vi "all-signals_counter-error-001.vi"() -> ()   [LabVIEW 2018]
uses:
  <vilib>/Platform/TimedLoop/XDataNode/timing_clust.ctl
  <vilib>/Platform/TimedLoop/XDataNode/nitl_modes.ctl
  <vilib>/Platform/TimedLoop/XDataNode/wakeup.ctl
  <vilib>/Analysis/baseanly.llb/Mean (DBL).vi
  <vilib>/platform/TimedLoop/XDataNode/XDataNode.xnode
  <vilib>/Analysis/NI_AALBase.lvlib
  <vilib>/Platform/TimedLoop/XDataNode/XDNodeRunTimeDep.lvlib
panel:
  in  "Clear Charts":bool
  in  "stop measurement (F)":bool caption="Stop measurements (F)"
  in  "Messzeit in ms":u32=100 min=10 max=1000 step=10
  in  "Tab Control":T1(tab)
  out "driving torque and counter":dynamicdata(graph)
  out "M_mech/N_motor":cluster{"Y":dbl[], "Y":dbl[]}[](graph)
  out "driving torque selected":dbl(graph)
  out "Motordrehzahl":dynamicdata(graph)
  out "Driving Torque gemittelt":dbl(graph)
  out "RPM and dn":dynamicdata(graph)
  out "Geschwindigkeit":dynamicdata(graph)
  out "Elektrische Leistung":waveform(dbl)(graph)
  out "RPM":dbl
  out "Bremsmoment":dynamicdata(graph)
  out "angular acc":dynamicdata(graph)
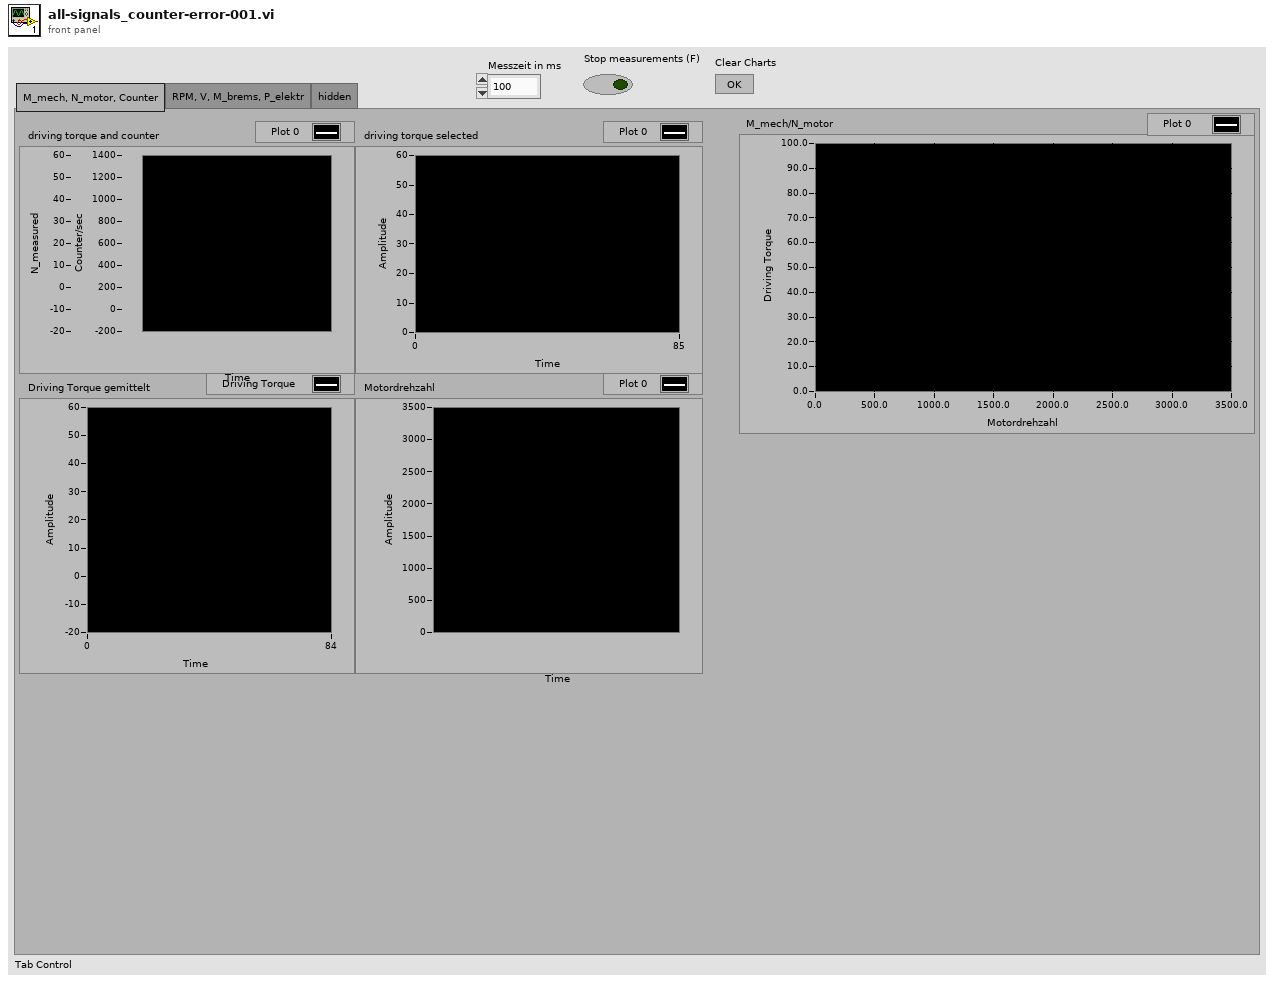
[diagram p1: front panel]
types:
  T1 = enum32{"M_mech, N_motor, Counter", "RPM, V, M_brems, P_elektr", "hidden"}
  T2 = typedef "XDNodeRunTimeDep.lvlib/timing_clust.ctl" = cluster{"Expected End [f-1]":u64, "Actual End [f-1]":u64, "Finished Late? [f-1]":bool, "Expected End [i-1]":u64, "Actual End [i-1]":u64, "Finished Late? [i-1]":bool, "Expected Start [i]":u64, "Actual Start [i]":u64, "Expected Start [f]":u64, "Actual Start [f]":u64, "Source Name":string, "Structure Name":string, "Period":i64, "Deadline":i64, "Offset":i64, "Start":i64, "Priority":i32, "Timeout":i32, "Mode":T3, "Wakeup Reason":T4, "Error":errorcluster, "Source Type":string, "Secondary Source Type":string, "Global End Time":u64, "Global Start Time":u64, "Frame Duration":u64, "Iteration Duration":u64, "Assigned CPU":i32, "I/O Scan Engine Mode":u32}
  T3 = typedef "XDNodeRunTimeDep.lvlib/nitl_modes.ctl" = enum32{"No Change", "Process missed periods, maintain original phase", "Discard missed periods, maintain original phase", "Process missed periods, ignore original phase", "Discard missed periods, ignore original phase"}
  T4 = typedef "XDNodeRunTimeDep.lvlib/wakeup.ctl" = enum32{"Normal", "Aborted", "Asynchronous wakeup", "Timing source error", "Timed loop error", "Timeout"}
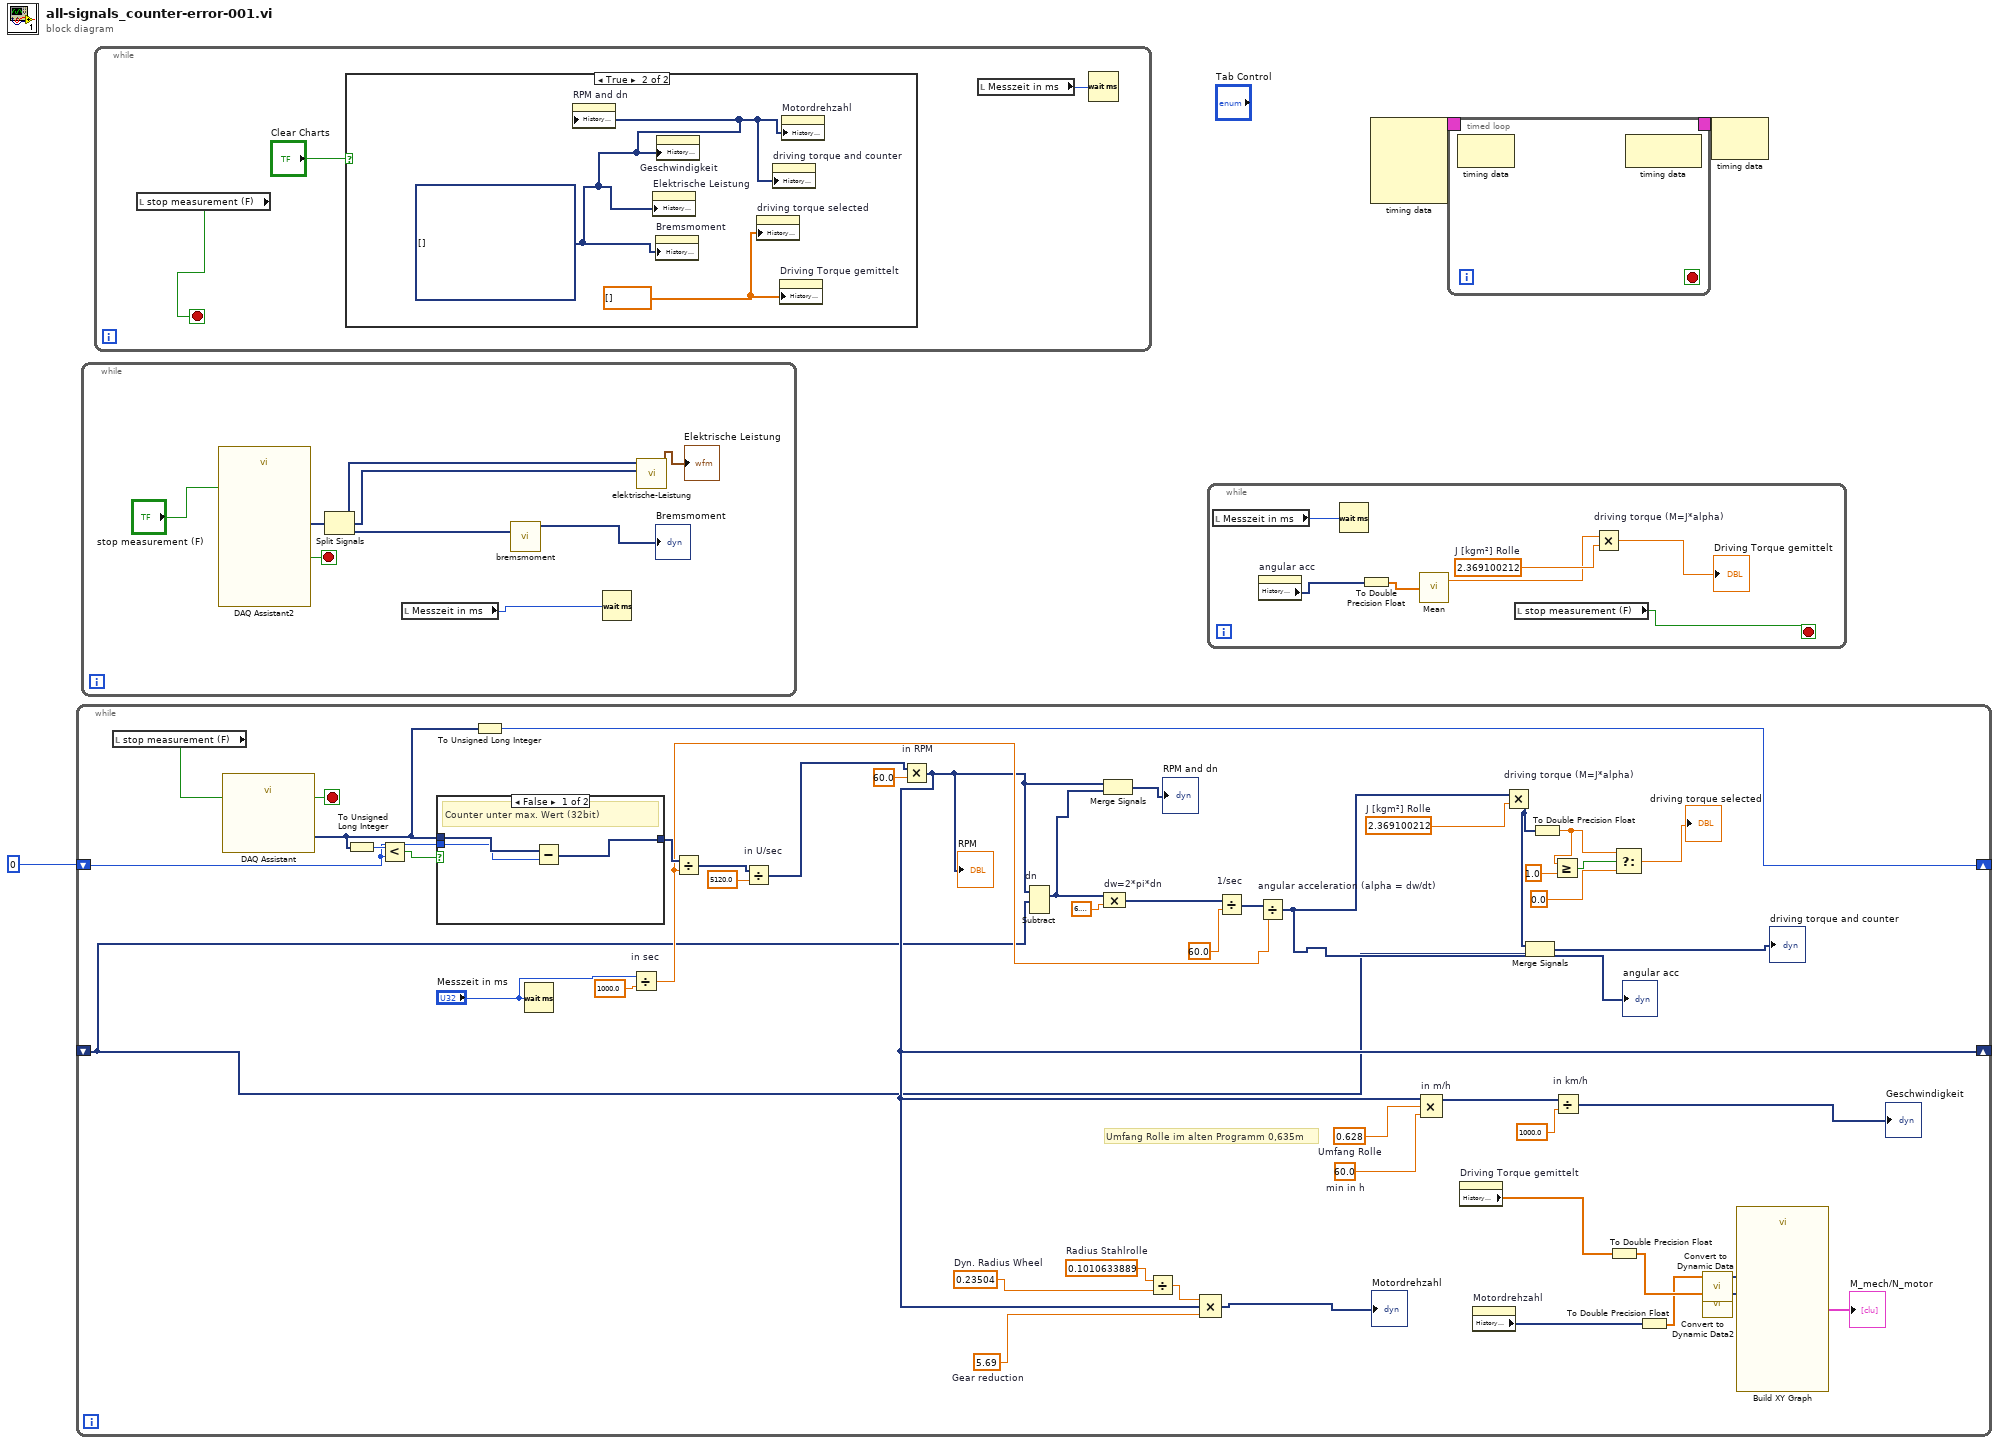
[diagram p0: block diagram]
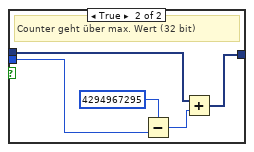
[diagram p2: hidden frame]
diagram:
  n1 = while {
    shift-right: [w50] -> _
    shift-left: u32 0 -> [w30]
    shift-right: [w25] -> _
    shift-left: _ -> [w6]
    stop <- w48 stop-if-true
    w22 = 2.369100212  # J [kgm²] Rolle
    w23 = 5.69  # Gear reduction
    w24 = 0.23504  # Dyn. Radius Wheel
    w27 = 0.1010633889  # Radius Stahlrolle
    w35 = 60.0  # min in h
    w34 = 0.628  # Umfang Rolle
    # "Umfang Rolle im alten Programm 0,635m"
    n2 = local read "stop measurement (F)"() -> (w5:bool)
    n3 = call "DAQ Assistant"("stop (F)"=w5) -> ("data"=w31:dynamicdata, "stopped"=w48:bool)  [unwired: 15 in, 2 out]
    n4 = To Unsigned Long Integer(number=w31) -> (unsigned 32bit integer=w49:u32)
    n5 = Less?(x=w49, y=w30) -> (x < y?=w52:bool)
    n6 = case shown="False" w52 {
      tunnel: w31 -> [w55 w57]
      tunnel: w30 -> [w54 w59]
      tunnel: [w53 w56] -> w45
      frame False {
        # "Counter unter max. Wert (32bit)"
        n7 = Subtract(x=w55, y=w54) -> (x-y=w53:dynamicdata)
      }
      frame True {
        # "Counter geht über max. Wert (32 bit)"
        n8 = Subtract(x=u32 4294967295, y=w59) -> (x-y=w58:u32)
        n9 = Add(x=w57, y=w58) -> (x+y=w56:dynamicdata)
      }
    }
    n10 = To Unsigned Long Integer(number=w31) -> (unsigned 32bit integer=w50:u32)
    n11 = Wait (ms)(milliseconds to wait="Messzeit in ms") -> ()  [unwired: 1 out]
    n12 = Divide "in sec"(x="Messzeit in ms", y=1000.0) -> (x/y=w38:dbl)
    n13 = Divide(x=w45, y=w38) -> (x/y=w44:dynamicdata)
    n14 = Divide "in U/sec"(x=w44, y=5120.0) -> (x/y=w33:dynamicdata)
    n15 = Multiply "in RPM"(x=w33, y=60.0) -> (x*y=w25:dynamicdata)
    "RPM" <- w25
    n16 = Subtract "dn"(1:w6, 2:w25) -> (0:w28:dynamicdata)  [unwired: 1 in, 1 out]
    n17 = Merge Signals(w25, w28) -> (→"RPM and dn":dynamicdata)
    n18 = Compound Arithmetic op=MULTIPLY "dw=2*pi*dn"(w28, 6.283185307179586) -> (w41:dynamicdata)
    n19 = Divide(x=w27, y=w24) -> (x/y=w26:dbl)
    n20 = Compound Arithmetic op=MULTIPLY(w26, w25, w23) -> (→"Motordrehzahl":dynamicdata)
    n21 = Divide "1/sec"(x=w41, y=60.0) -> (x/y=w39:dynamicdata)
    n22 = Divide "angular acceleration (alpha = dw/dt)"(x=w39, y=w38) -> (x/y=w8:dynamicdata)
    "angular acc" <- w8
    n23 = Compound Arithmetic op=MULTIPLY "in m/h"(w25, w34, w35) -> (w36:dynamicdata)
    n24 = property on="Driving Torque gemittelt" class="WFChart (strict)"() -> ("History Data"=w4:dbl[])  [unwired: 2 in, 2 out]
    n25 = property on="Motordrehzahl" class="WFChart (strict)"() -> ("History Data"=w16:dynamicdata[])  [unwired: 2 in, 2 out]
    n26 = Multiply "driving torque (M=J*alpha)"(x=w8, y=w22) -> (x*y=w14:dynamicdata)
    n27 = Merge Signals(w14, w6) -> (→"driving torque and counter":dynamicdata)
    n28 = To Double Precision Float(number=w14) -> (double precision float=w13:dbl)
    n29 = Greater Or Equal?(x=w13, y=1.0) -> (x >= y?=w11:bool)
    n30 = Divide "in km/h"(x=w36, y=1000.0) -> (x/y=→"Geschwindigkeit":dynamicdata)
    n31 = To Double Precision Float(number=w4) -> (double precision float=w21:dbl[])
    n32 = Select(t=w13, s=w11, f=0.0) -> (s? t:f=→"driving torque selected":dbl)
    n33 = To Double Precision Float(number=w16) -> (double precision float=w18:dbl[])
    n34 = call "Convert to Dynamic Data"("Array"=w18) -> ("Dynamic Data Type"=w19:dynamicdata)  [unwired: 3 in]
    n35 = call "Convert to Dynamic Data2"("Array"=w21) -> ("Dynamic Data Type"=w20:dynamicdata)  [unwired: 3 in]
    n36 = call "Build XY Graph"("Y Input"=w20, "X Input"=w19) -> ("XY Graph"=→"M_mech/N_motor":cluster{"X":dbl[], "Y":dbl[]}[])  [unwired: 8 in, 1 out]
  }
  n37 = while {
    stop <- w64 stop-if-true
    n38 = call "DAQ Assistant2"("stop (F)"="stop measurement (F)") -> ("data"=w65:dynamicdata, "stopped"=w64:bool)  [unwired: 15 in, 2 out]
    n39 = Split Signals(w65) -> (w69:dynamicdata, w68:dynamicdata, w67:dynamicdata)  [unwired: 3 in]
    n40 = local read "Messzeit in ms"() -> (w61:u32)
    n41 = call "bremsmoment.vi"("Dynamic Data in"=w67) -> ("Dynamic Data out"=→"Bremsmoment":dynamicdata)  [unwired: 10 in]
    n42 = Wait (ms)(milliseconds to wait=w61) -> ()  [unwired: 1 out]
    n43 = call "elektrische-Leistung.vi"("Dynamic Data"=w68, "Dynamic Data 2"=w69) -> ("Elektrische Leistung"=→"Elektrische Leistung":waveform(dbl))  [unwired: 9 in]
  }
  n44 = while {
    stop <- w70 stop-if-true
    n45 = local read "stop measurement (F)"() -> (w70:bool)
    n46 = case shown="True" "Clear Charts" {
      frame False {
      }
      frame True {
        w74 = dbl[] [] ("History Data")
        w73 = dynamicdata[] [] ("History Data")
        n47 = property on="RPM and dn" class="WFChart (strict)"("History Data"=w73) -> ()  [unwired: 2 in, 2 out]
        n48 = property on="Elektrische Leistung" class="WFChart (strict)"("History Data"=w73) -> ()  [unwired: 2 in, 2 out]
        n49 = property on="Bremsmoment" class="WFChart (strict)"("History Data"=w73) -> ()  [unwired: 2 in, 2 out]
        n50 = property on="Geschwindigkeit" class="WFChart (strict)"("History Data"=w73) -> ()  [unwired: 2 in, 2 out]
        n51 = property on="driving torque selected" class="WFChart (strict)"("History Data"=w74) -> ()  [unwired: 2 in, 2 out]
        n52 = property on="driving torque and counter" class="WFChart (strict)"("History Data"=w73) -> ()  [unwired: 2 in, 2 out]
        n53 = property on="Driving Torque gemittelt" class="WFChart (strict)"("History Data"=w74) -> ()  [unwired: 2 in, 2 out]
        n54 = property on="Motordrehzahl" class="WFChart (strict)"("History Data"=w73) -> ()  [unwired: 2 in, 2 out]
      }
    }
    n55 = local read "Messzeit in ms"() -> (w71:u32)
    n56 = Wait (ms)(milliseconds to wait=w71) -> ()  [unwired: 1 out]
  }
  n57 = while {
    stop <- w75 stop-if-true
    w80 = 2.369100212  # J [kgm²] Rolle
    n58 = local read "Messzeit in ms"() -> (w76:u32)
    n59 = property on="angular acc" class="WFChart (strict)"() -> ("History Data"=w77:dynamicdata[])  [unwired: 2 in, 2 out]
    n60 = Wait (ms)(milliseconds to wait=w76) -> ()  [unwired: 1 out]
    n61 = To Double Precision Float(number=w77) -> (double precision float=w81:dbl[])
    n62 = call-poly <vilib>:"Mean.vi"("X"=w81) -> ("mean"=w78:dbl)  [unwired: 1 out]
    n63 = local read "stop measurement (F)"() -> (w75:bool)
    n64 = Multiply "driving torque (M=J*alpha)"(x=w78, y=w80) -> (x*y=→"Driving Torque gemittelt":dbl)
  }
  n65 = node-c288() -> (w2:T2)  [unwired: 4 in]
  n66 = timed-loop {
    timing: w2 -> [_]
    timing-out: [_] -> w1
    stop <- _ stop-if-true
    n67 = node-c288() -> ()  [unwired: 1 in, 1 out]
    n68 = node-c288() -> ()  [unwired: 1 in, 1 out]
  }
  n69 = node-c288(w1) -> ()  [unwired: 1 out]
